vi "wait -- subVI.vi"(2 "milliseconds to wait":u32=100, 5 "error in (no error)":errorcluster) -> (1 "error out":errorcluster)   [LabVIEW 2020]
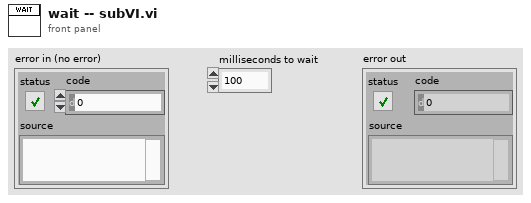
[diagram p1: front panel]
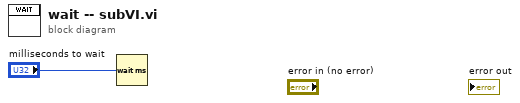
[diagram p0: block diagram]
diagram:
  n1 = Wait (ms)(milliseconds to wait="milliseconds to wait") -> ()  [unwired: 1 out]
